vi "EventExeIntDouble.vi"(8 "error in (no error)":errorcluster, 10 "Event Registration Refnum In":refnum<event-registration>, 11 "Device In":i32) -> (0 "error out":errorcluster, 1 "index":i32, 2 "Event Registration Refnum Out":refnum<event-registration>, 3 "Device Out":i32, 4 "acceleration":dbl, 5 "Event?":bool)   [LabVIEW 2012]
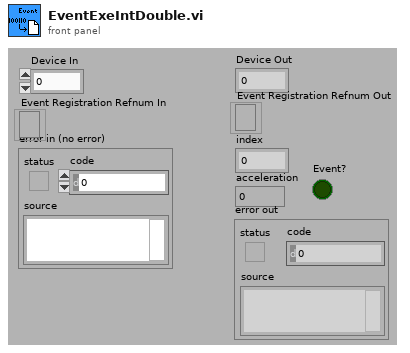
[diagram p1: front panel]
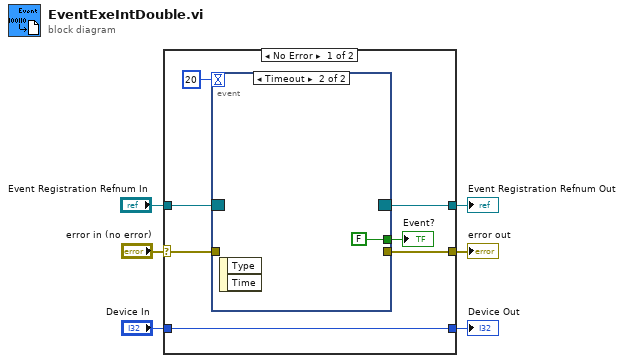
[diagram p0: block diagram]
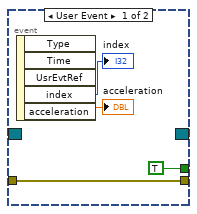
[diagram p2: hidden frame]
diagram:
  n1 = case shown="No Error" "error in (no error)" {
    selector: "error in (no error)" -> [w13 w21]
    tunnel: [w12 w21] -> w5
    tunnel: "Device In" -> [w11 w20]
    tunnel: [w11 w20] -> w3
    tunnel: [w10 w19] -> w2
    tunnel: "Event Registration Refnum In" -> [w9 w19]
    frame No Error {
      n2 = event shown="[1] Timeout" {
        selector: w9 -> [_ _]
        dyn-events: [_ _] -> w10
        timeout: 20 -> [_ _]
        tunnel: w13 -> [w15 _]
        tunnel: [w15 _] -> w12
        tunnel: [TRUE ("stop") FALSE ("stop")] -> w7
        event User Event {
          n3 = event-data() -> ("index"=→"index":i32, "acceleration"=→"acceleration":dbl)  [unwired: 1 in, 3 out]
        }
        event Timeout {
          n4 = event-data() -> ()  [unwired: 1 in, 2 out]
        }
      }
      "Event?" <- w7
    }
    frame Error {
    }
  }
  "Device Out" <- w3
  "error out" <- w5
  "Event Registration Refnum Out" <- w2
